vi "Example Publisher.vi"() -> ()   [LabVIEW 2021]
uses:
  TCP_Streamer_Publisher/Typedef/State.ctl
  TCP_Streamer_Publisher/Typedef/Configuration.ctl
  TCP_Streamer_Publisher/TCP_Streamer_Publisher.lvclass/TCP_Streamer_Publisher.ctl
  TCP_Streamer_Publisher/TCP_Streamer_Publisher.lvclass
panel:
  out "Timeout":bool
  out "port":u16
  out "remote address":string
  out "remote port":u16
  in  "Configuration":T1={"IP Address"="localhost", "port"=0}
  in  "delay (ms)":u32=100
  out "State":T2=enum."Listening"
  in  "stop":bool
  out "error out":errorcluster
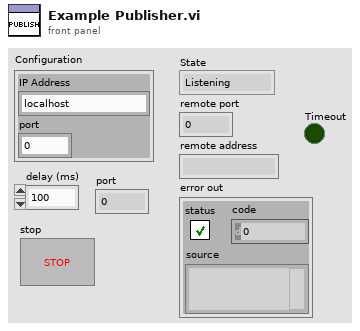
[diagram p1: front panel]
types:
  T1 = typedef "TCP_Streamer_Publisher.lvclass/Configuration.ctl" = cluster{"IP Address":string, "port":u16}
  T2 = typedef "TCP_Streamer_Publisher.lvclass/State.ctl" = enum16{"Stopped", "Listening", "Ready for Data", "Ready to Send", "Sending"}
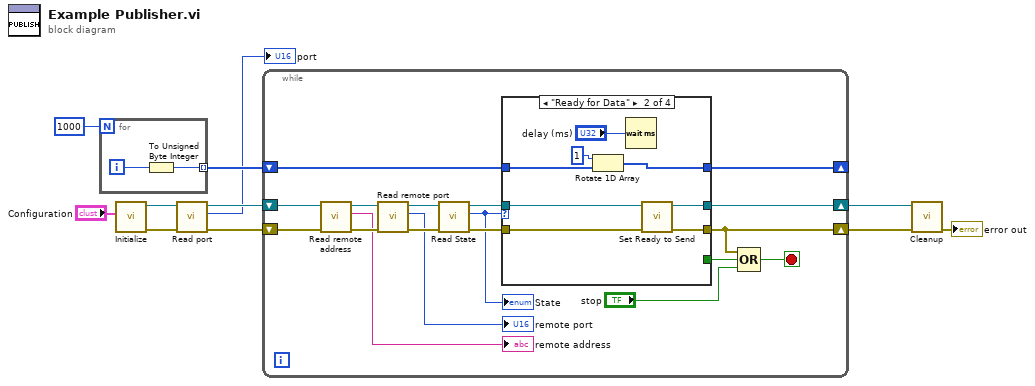
[diagram p0: block diagram]
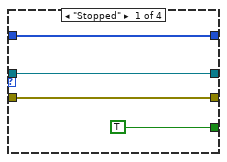
[diagram p2: hidden frame]
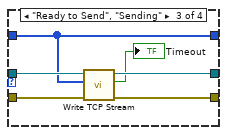
[diagram p3: hidden frame]
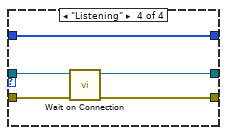
[diagram p4: hidden frame]
diagram:
  n1 = for {
    N: 1000 -> [_]
    tunnel: [w12] -> w7 mode=indexing
    i -> [w13]
    n2 = To Unsigned Byte Integer(number=w13) -> (unsigned 8bit integer=w12:u8)
  }
  n3 = call "Initialize.vi"("Configuration"="Configuration") -> ("error out"=w4:errorcluster, "TCP_Streamer out"=w5:refnum<class "TCP_Streamer_Publisher.lvclass">)  [unwired: 9 in]
  n4 = call "Read port.vi"("error in (no error)"=w4, "TCP_Streamer in"=w5) -> ("error out"=w2:errorcluster, "port"=→"port":u16, "TCP_Streamer out"=w3:refnum<class "TCP_Streamer_Publisher.lvclass">)  [unwired: 7 in]
  n5 = while {
    shift-right: [w17] -> w11
    shift-left: w3 -> [w21]
    shift-right: [w16] -> w10
    shift-left: w2 -> [w20]
    shift-right: [w24] -> _
    shift-left: w7 -> [w25]
    stop <- w26 stop-if-true
    n6 = call "Read remote address.vi"("error in (no error)"=w20, "TCP_Streamer in"=w21) -> ("error out"=w19:errorcluster, "remote address"=→"remote address":string, "TCP_Streamer out"=w22:refnum<class "TCP_Streamer_Publisher.lvclass">)  [unwired: 7 in]
    n7 = call "Read remote port.vi"("error in (no error)"=w19, "TCP_Streamer in"=w22) -> ("error out"=w18:errorcluster, "remote port"=→"remote port":u16, "TCP_Streamer out"=w23:refnum<class "TCP_Streamer_Publisher.lvclass">)  [unwired: 7 in]
    n8 = call "Read State.vi"("error in (no error)"=w18, "TCP_Streamer in"=w23) -> ("error out"=w30:errorcluster, "State"=w29:T2, "TCP_Streamer out"=w31:refnum<class "TCP_Streamer_Publisher.lvclass">)  [unwired: 7 in]
    "State" <- w29
    n9 = case shown="\"Ready for Data\"" w29 {
      tunnel: [w35 w41 w46 w54] -> w17
      tunnel: [w34 w42 w47 w53] -> w16
      tunnel: w31 -> [w35 w40 w49 w52]
      tunnel: w30 -> [w34 w43 w48 w51]
      tunnel: [TRUE _ _ _] -> w28
      tunnel: w25 -> [w32 w39 w45 w50]
      tunnel: [w32 w38 w45 w50] -> w24
      frame "Stopped" {
      }
      frame "Ready for Data" {
        n10 = Rotate 1D Array(1:w39, 2:1 ("n")) -> (0:w38:u8[])
        n11 = Wait (ms)(milliseconds to wait="delay (ms)") -> ()  [unwired: 1 out]
        n12 = call "Set Ready to Send.vi"("error in (no error)"=w43, "TCP_Streamer in"=w40) -> ("error out"=w42:errorcluster, "TCP_Streamer out"=w41:refnum<class "TCP_Streamer_Publisher.lvclass">)  [unwired: 8 in]
      }
      frame "Ready to Send", "Sending" {
        n13 = call "Write TCP Stream.vi"("error in (no error)"=w48, "Data"=w45, "TCP_Streamer in"=w49) -> ("error out"=w47:errorcluster, "Timeout"=→"Timeout":bool, "TCP_Streamer out"=w46:refnum<class "TCP_Streamer_Publisher.lvclass">)  [unwired: 6 in]
      }
      frame "Listening" {
        n14 = call "Wait on Connection.vi"("error in (no error)"=w51, "TCP_Streamer in"=w52) -> ("error out"=w53:errorcluster, "TCP_Streamer out"=w54:refnum<class "TCP_Streamer_Publisher.lvclass">)  [unwired: 8 in]
      }
    }
    n15 = Compound Arithmetic op=OR(w16, w28, "stop") -> (w26:bool)
  }
  n16 = call "Cleanup.vi"("error in (no error)"=w10, "TCP_Streamer in"=w11) -> ("error out"=→"error out":errorcluster)  [unwired: 8 in, 1 out]
